vi "Rotating Vectors.vi"() -> ()   [LabVIEW 2015]
uses:
  <vilib>/Analysis/1siggen.llb/Ramp Pattern by Samples.vi
  <vilib>/Analysis/2dsp.llb/Complex FFT.vi
  <vilib>/Analysis/2dsp.llb/Real FFT.vi
  Sub - Arrow Point Calculate.vi
  <vilib>/Analysis/NI_AALPro.lvlib
  <vilib>/Analysis/NI_AALBase.lvlib
panel:
  in  "Message Amplitude":dbl=0.5
  in  "DC Offset":dbl
  in  "RF Frequency":dbl
  in  "Message Frequency":dbl=0.2 step=0.1
  in  "stop":bool
  in  "vi path":path
  in  "Vertical Load Button":bool
  in  "Vertical Pause Button":bool
  in  "Upconvert Baseband":bool=TRUE
  out "Vector Graph":cluster{"z vector":cdb[]}[](graph)=[{"z vector"=[0.0+0.0i, 0.20656463842372266-0.4553361946439979i, 0.21632021300842424-0.355813188436778i, 0.20656463842372266-0.4553361946439979i, 0.12525297407962463-0.3971261161215226i, 0.20656463842372266-0.4553361946439979i]}, {"z vector"=[0.0+0.0i, 0.20656463842372266+0.4553361946439979i, 0.1252529740796247+0.3971261161215225i, 0.20656463842372266+0.4553361946439979i, 0.21632021300842427+0.355813188436778i, 0.20656463842372266+0.4553361946439979i]}, {"z vector"=[0.0+0.0i, 0.4131292768474453+0.0i, 0.32652673646900143+0.05000000000000002i, 0.4131292768474453+0.0i, 0.3265267364690015-0.050000000000000044i, 0.4131292768474453+0.0i]}, {"z vector"=[0.0+0.0i, 0.0+0.0i, nan+nani, 0.0+0.0i, nan+nani, 0.0+0.0i]}, {"z vector"=[0.0+0.0i, 0.4131292768474453+0.0i, 0.32652673646900143+0.05000000000000002i, 0.4131292768474453+0.0i, 0.3265267364690015-0.050000000000000044i, 0.4131292768474453+0.0i]}, {"z vector"=[0.0+0.0i, 0.4131292768474453+0.0i, 0.32652673646900143+0.05000000000000002i, 0.4131292768474453+0.0i, 0.3265267364690015-0.050000000000000044i, 0.4131292768474453+0.0i]}, {"z vector"=[0.4131292768474453+0.0i, 0.4131292768474453+0.0i, nan+nani, 0.4131292768474453+0.0i, nan+nani, 0.4131292768474453+0.0i]}, {"z vector"=[0.0+0.0i, 1.0+0.0i, 0.9133974596215562+0.05000000000000002i, 1.0+0.0i, 0.9133974596215562-0.050000000000000044i, 1.0+0.0i]}]
  out "Time Domain":cluster{dbl, dbl, dbl}(graph)={0.4131292768474453, 0.4131292768474453, 1.0}
  out "Vector Sum Frequency Response":dbl[][](graph)
  out "Individual Vectors":dbl[][](graph)
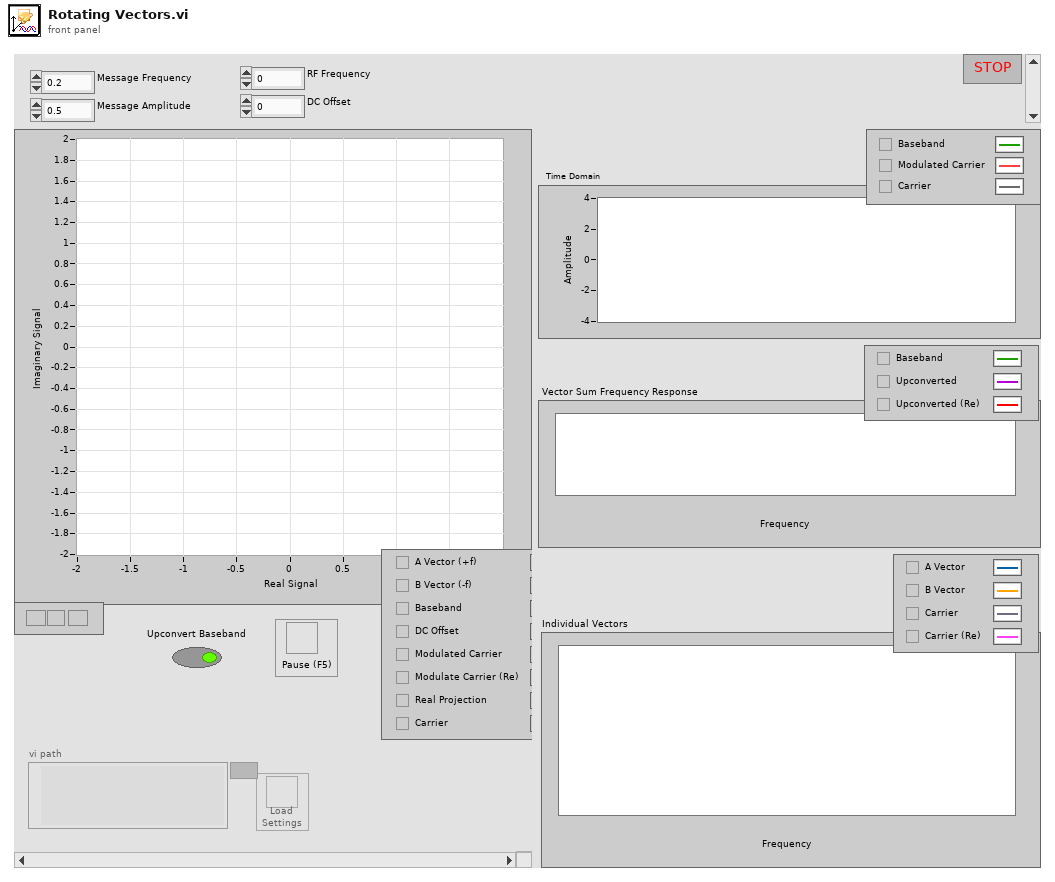
[diagram p1: front panel]
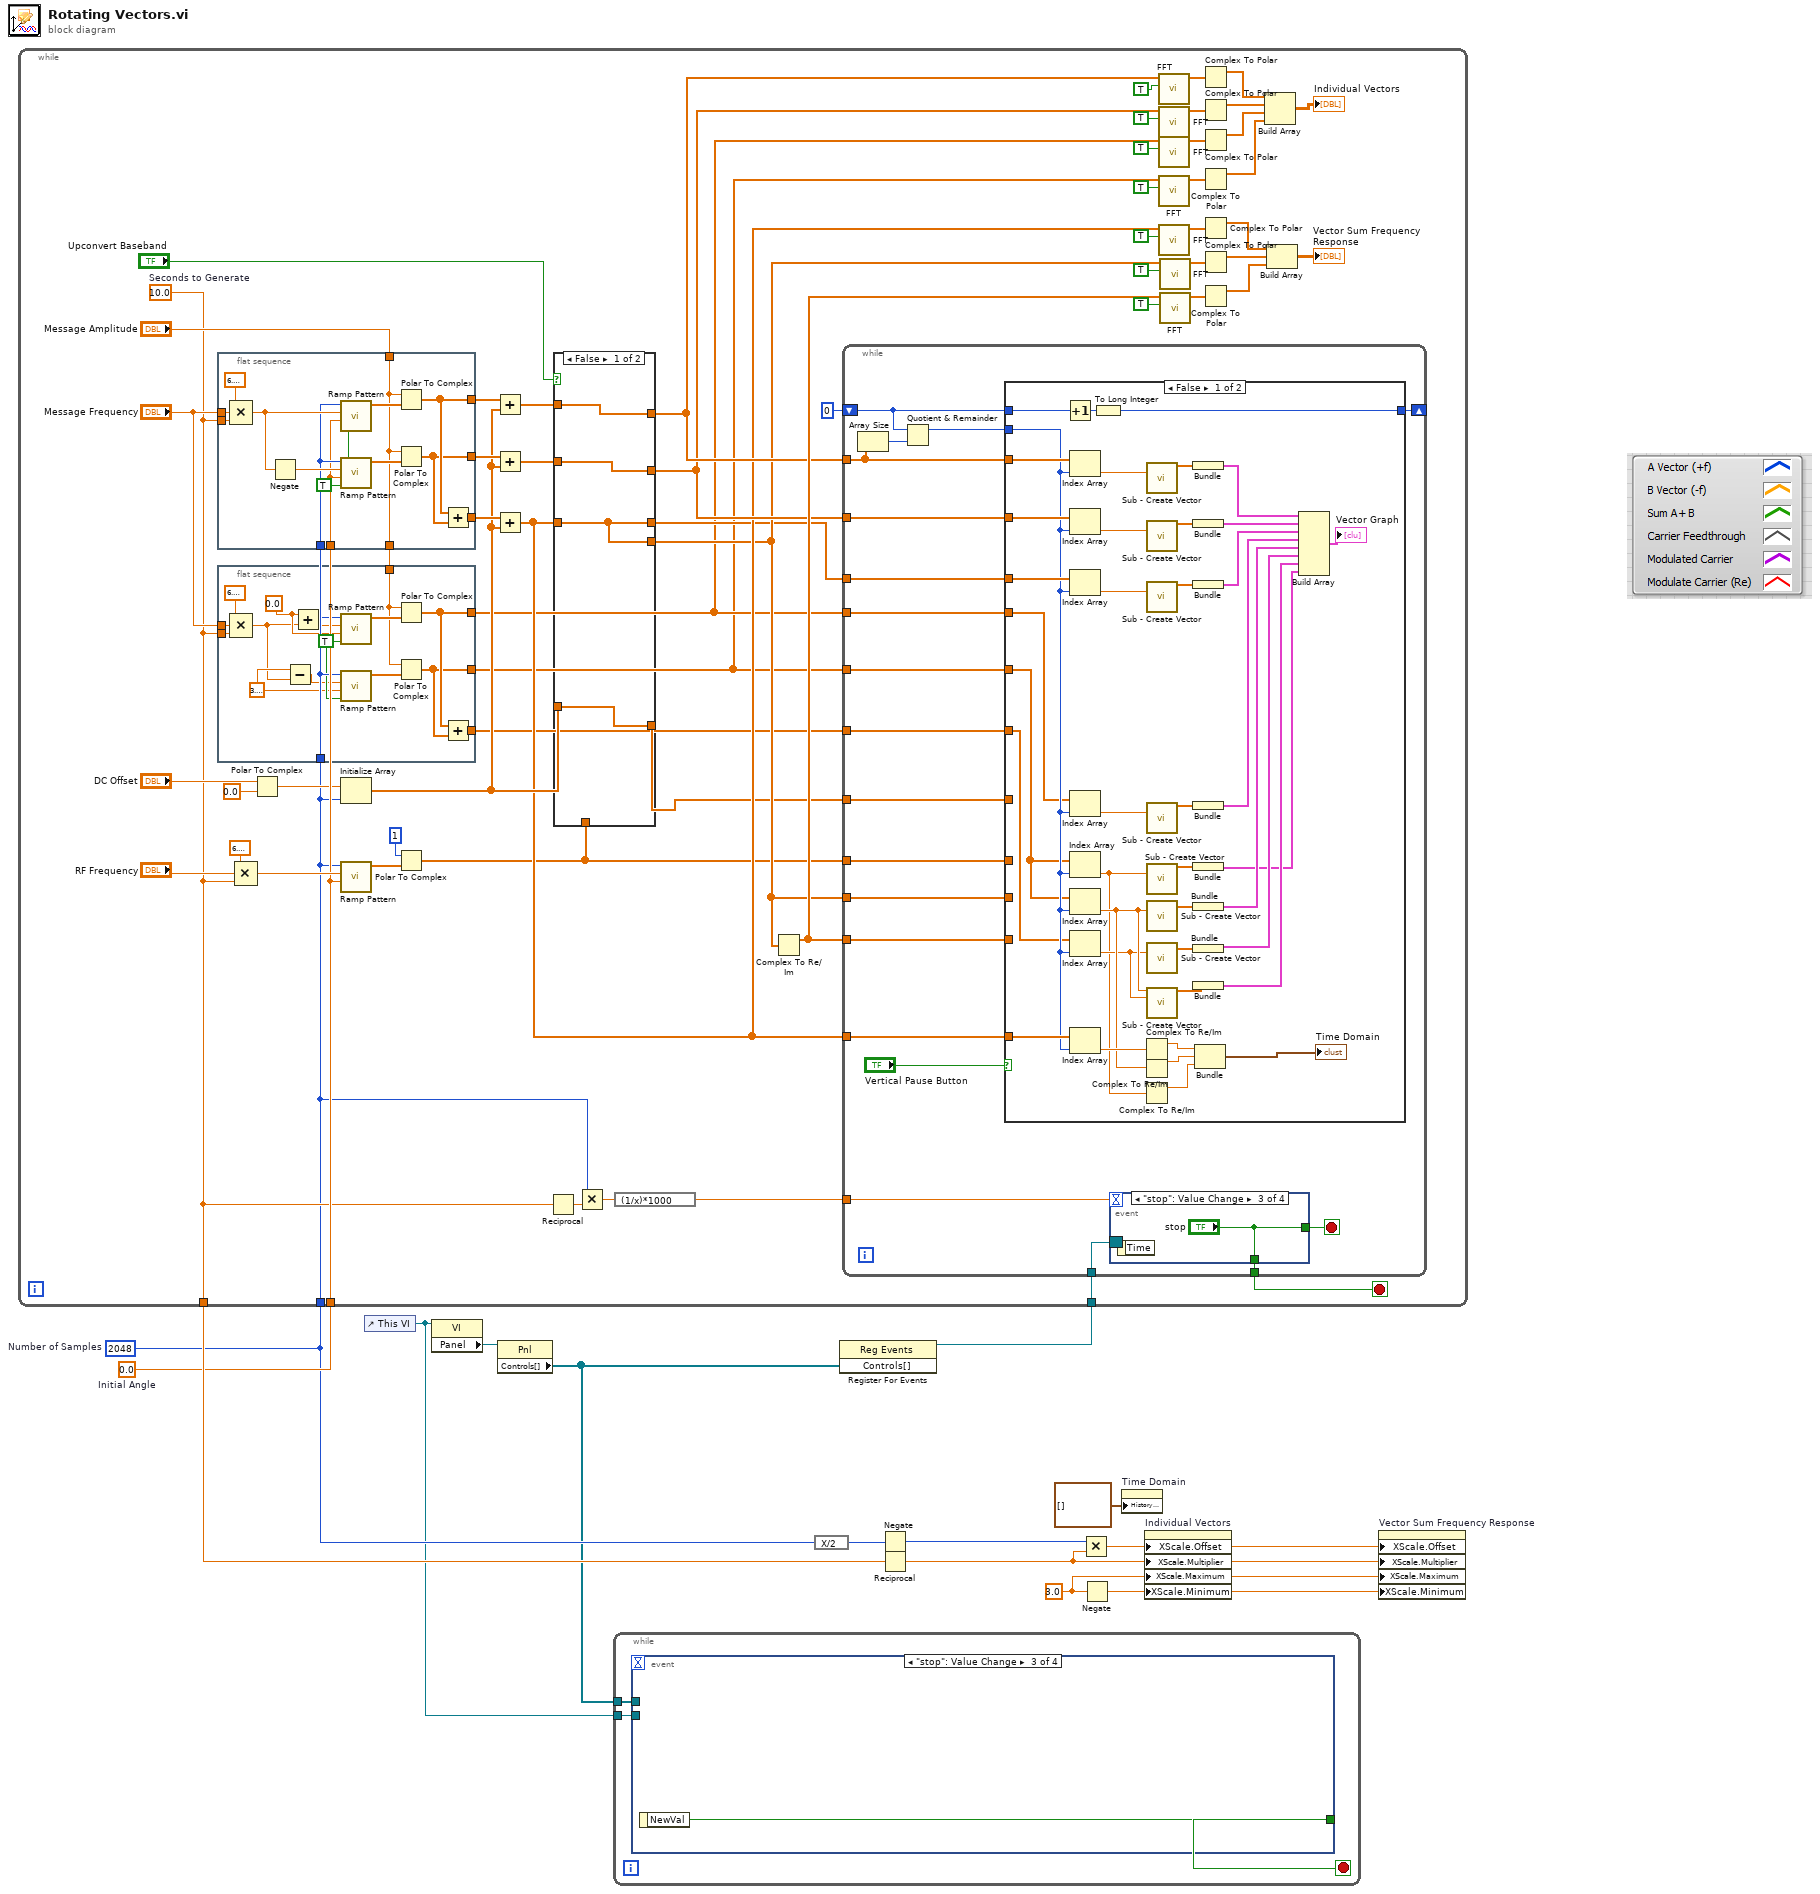
[diagram p0: block diagram]
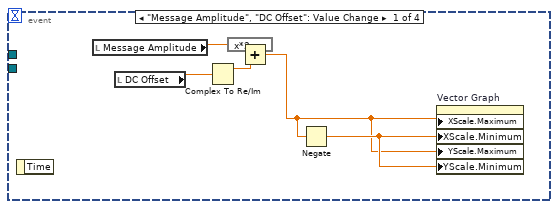
[diagram p2: hidden frame]
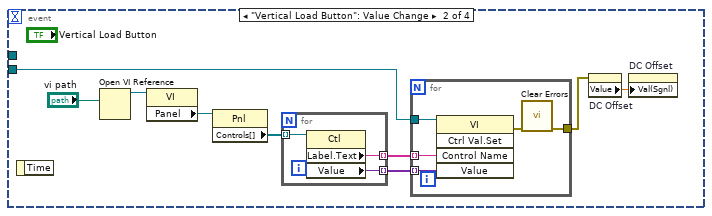
[diagram p3: hidden frame]
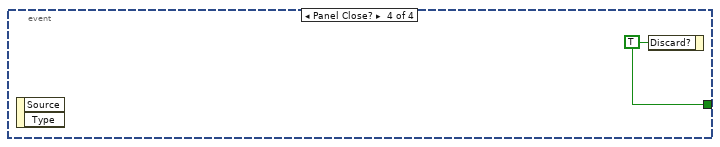
[diagram p4: hidden frame]
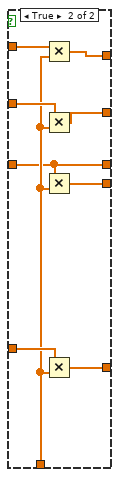
[diagram p5: hidden frame]
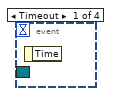
[diagram p7: hidden frame]
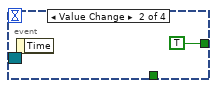
[diagram p8: hidden frame]
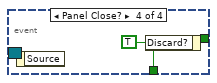
[diagram p9: hidden frame]
diagram:
  w4 = 2048  # Number of Samples
  w5 = 0.0  # Initial Angle
  w11 = 3.0 ("X Scale.Range:Maximum")
  n1 = control-ref of="This VI"() -> (w1:refnum<vi>)
  n2 = property class="VI"(reference=w1) -> ("Panel"=w7:refnum<vi>)  [unwired: 1 in, 2 out]
  n3 = property class="Pnl"(reference=w7) -> ("Controls[]"=w2:refnum<vi>[])  [unwired: 1 in, 2 out]
  n4 = while {
    tunnel: w2 -> [w16]
    tunnel: w1 -> [w15]
    stop <- w17 stop-if-true
    n5 = event shown="[2] \"stop\": Value Change" {
      selector: _ -> [_ _ _ _]
      dyn-events: _ -> [_ _ _ _]
      timeout: _ -> [_ _ _ _]
      tunnel: [_ _ w41 w42] -> w17
      tunnel: w16 -> [_ _ _ _]
      tunnel: w15 -> [_ w29 _ _]
      event "Message Amplitude", "DC Offset": Value Change {
        n6 = event-data() -> ()  [unwired: 1 in, 1 out]
        n7 = local read "Message Amplitude"() -> (w21:dbl)
        n8 = local read "DC Offset"() -> (w22:dbl)
        n9 = Complex To Re/Im(x + iy=w22) -> (x=w19:dbl)  [unwired: 1 out]
        n10 = expression code="x*2"(w21) -> (w18:dbl)
        n11 = Add(x=w18, y=w19) -> (x+y=w20:dbl)
        n12 = Negate(x=w20) -> (-x=w23:dbl)
        n13 = property on="Vector Graph" class="XYGraph (strict)"("XScale.Maximum"=w20, "XScale.Minimum"=w23, "YScale.Maximum"=w20, "YScale.Minimum"=w23) -> ()  [unwired: 2 in, 2 out]
      }
      event "Vertical Load Button": Value Change {
        n14 = event-data() -> ()  [unwired: 1 in, 1 out]
        n15 = Open VI Reference(vi path="vi path") -> (vi reference=w31:refnum<vi>)  [unwired: 5 in, 1 out]
        n16 = property class="VI"(reference=w31) -> ("Panel"=w32:refnum<vi>)  [unwired: 1 in, 2 out]
        n17 = property class="Pnl"(reference=w32) -> ("Controls[]"=w30:refnum<vi>[])  [unwired: 1 in, 2 out]
        n18 = for {
          tunnel: w30 -> [w40] mode=indexing
          tunnel: [w39] -> w28 mode=indexing
          tunnel: [w38] -> w27 mode=indexing
          n19 = property class="Ctl"(reference=w40) -> ("Label.Text"=w39:string, "Value"=w38:variant)  [unwired: 1 in, 2 out]
        }
        n20 = for {
          tunnel: w29 -> [w37]
          tunnel: w28 -> [w36] mode=indexing
          tunnel: w27 -> [w35] mode=indexing
          tunnel: [w33] -> w24
          n21 = invoke class="VI" method="Ctrl Val.Set"(reference=w37, "Control Name"=w36, "Value"=w35) -> (error out=w34:errorcluster)  [unwired: 2 in, 4 out]
          n22 = call <vilib>:"Clear Errors.vi"("error in (no error)"=w34) -> ("error out"=w33:errorcluster)  [unwired: 5 in, 1 out]
        }
        n23 = property on="DC Offset" class="DigNum (strict)"(error in=w24) -> ("Value"=w25:dbl)  [unwired: 1 in, 2 out]
        n24 = property on="DC Offset" class="DigNum (strict)"("Val(Sgnl)"=w25) -> ()  [unwired: 2 in, 2 out]
      }
      event "stop": Value Change {
        n25 = event-data() -> ("NewVal"=w41:bool)  [unwired: 1 in]
      }
      event Panel Close? {
        w42 = TRUE ("Discard?")
        n26 = event-data() -> ()  [unwired: 1 in, 2 out]
        n27 = event-data("Discard?"=w42) -> ()  [unwired: 1 in, 1 out]
      }
    }
  }
  n28 = expression code="X/2"(w4) -> (w13:i32)
  n29 = register-events(w2) -> (reference out=w6:refnum<event-registration>)  [unwired: 2 in, 1 out]
  n30 = while {
    tunnel: [w49] -> w8
    tunnel: w4 -> [w48]
    tunnel: w6 -> [w81]
    tunnel: w5 -> [w72]
    stop <- w79 stop-if-true
    w49 = 10.0  # Seconds to Generate
    n31 = flat-sequence {
      tunnel: "Message Frequency" -> [w132]
      tunnel: [w127] -> w83
      tunnel: [w126] -> w82
      tunnel: w48 -> [w125]
      tunnel: "Message Amplitude" -> [w121]
      tunnel: w49 -> [w124]
      tunnel: [w123] -> w73
      tunnel: w72 -> [w122]
      tunnel: [w121] -> w46
      frame #0 {
        w120 = TRUE ("exclude end?")
        n32 = Compound Arithmetic op=MULTIPLY(6.283185307179586, w132, w124) -> (w128:dbl)
        n33 = Negate(x=w128) -> (-x=w129:dbl)
        n34 = call-poly <vilib>:"Ramp Pattern.vi"("exclude end?"=w120, "start"=w122, "end"=w128, "samples"=w125) -> ("Ramp Pattern"=w131:dbl[])  [unwired: 6 in, 1 out]
        n35 = call-poly <vilib>:"Ramp Pattern.vi"("exclude end?"=w120, "start"=w122, "end"=w129, "samples"=w125) -> ("Ramp Pattern"=w130:dbl[])  [unwired: 6 in, 1 out]
        n36 = Polar To Complex(1:w131, 2:w121) -> (0:w127:cdb[])
        n37 = Polar To Complex(1:w130, 2:w121) -> (0:w126:cdb[])
        n38 = Add(x=w127, y=w126) -> (x+y=w123:cdb[])
      }
    }
    n39 = flat-sequence {
      tunnel: [w116] -> w44
      tunnel: [w115] -> w43
      tunnel: w49 -> [w114]
      tunnel: [w113] -> w47
      tunnel: "Message Frequency" -> [w112]
      tunnel: w48 -> [w111]
      tunnel: w46 -> [w110]
      frame #0 {
        w106 = 3.141592653589793
        w107 = 0.0 ("start")
        w109 = TRUE ("exclude end?")
        n40 = Compound Arithmetic op=MULTIPLY(6.283185307179586, w112, w114) -> (w105:dbl)
        n41 = Subtract(x=w106, y=w105) -> (x-y=w104:dbl)
        n42 = Add(x=w107, y=w105) -> (x+y=w108:dbl)
        n43 = call-poly <vilib>:"Ramp Pattern.vi"("exclude end?"=w109, "start"=w107, "end"=w108, "samples"=w111) -> ("Ramp Pattern"=w118:dbl[])  [unwired: 6 in, 1 out]
        n44 = call-poly <vilib>:"Ramp Pattern.vi"("exclude end?"=w109, "start"=w106, "end"=w104, "samples"=w111) -> ("Ramp Pattern"=w117:dbl[])  [unwired: 6 in, 1 out]
        n45 = Polar To Complex(1:w118, 2:w110) -> (0:w116:cdb[])
        n46 = Polar To Complex(1:w117, 2:w110) -> (0:w115:cdb[])
        n47 = Add(x=w116, y=w115) -> (x+y=w113:cdb[])
      }
    }
    n48 = Compound Arithmetic op=MULTIPLY(6.283185307179586, "RF Frequency", w49) -> (w84:dbl)
    n49 = Polar To Complex(1:0.0 ("theta"), 2:"DC Offset") -> (0:w58:cdb)
    n50 = Initialize Array(w58, w48) -> (w62:cdb[])
    n51 = call-poly <vilib>:"Ramp Pattern.vi"("start"=w72, "end"=w84, "samples"=w48) -> ("Ramp Pattern"=w90:dbl[])  [unwired: 7 in, 1 out]
    n52 = Polar To Complex(1:w90, 2:1) -> (0:w52:cdb[])
    n53 = Add(x=w83, y=w62) -> (x+y=w67:cdb[])
    n54 = Add(x=w82, y=w62) -> (x+y=w66:cdb[])
    n55 = Add(x=w73, y=w62) -> (x+y=w61:cdb[])
    n56 = Reciprocal(x=w49) -> (1/x=w98:dbl)
    n57 = case shown="False" "Upconvert Baseband" {
      tunnel: w67 -> [w135 w146]
      tunnel: w66 -> [w136 w145]
      tunnel: w62 -> [w137 w144]
      tunnel: w61 -> [w134 w138]
      tunnel: w52 -> [_ w143]
      tunnel: [w137 w142] -> w55
      tunnel: [w134 w141] -> w60
      tunnel: [w136 w140] -> w63
      tunnel: [w135 w139] -> w64
      tunnel: [w134 w138] -> w56
      frame False {
      }
      frame True {
        n58 = Multiply(x=w146, y=w143) -> (x*y=w139:cdb[])
        n59 = Multiply(x=w145, y=w143) -> (x*y=w140:cdb[])
        n60 = Multiply(x=w138, y=w143) -> (x*y=w141:cdb[])
        n61 = Multiply(x=w144, y=w143) -> (x*y=w142:cdb[])
      }
    }
    n62 = Multiply(x=w48, y=w98) -> (x*y=w99:dbl)
    n63 = expression code="(1/x)*1000"(w99) -> (w103:dbl)
    n64 = Complex To Re/Im(x + iy=w60) -> (x=w68:dbl[])  [unwired: 1 out]
    n65 = while {
      tunnel: w64 -> [w157]
      tunnel: w103 -> [w162]
      tunnel: w63 -> [w166]
      tunnel: w56 -> [w165]
      tunnel: w60 -> [w164]
      tunnel: w55 -> [w163]
      tunnel: w81 -> [w158]
      tunnel: [w160] -> w79
      tunnel: w68 -> [w159]
      tunnel: w61 -> [w155]
      shift-right: [w152] -> _
      shift-left: 0 -> [w153]
      tunnel: w52 -> [w150]
      tunnel: w44 -> [w149]
      tunnel: w43 -> [w148]
      tunnel: w47 -> [w147]
      stop <- w161 stop-if-true
      n66 = Array Size(array=w157) -> (size(s)=w156:i32)
      n67 = Quotient & Remainder(x=w153, y=w156) -> (x-y*floor(x/y)=w154:i32)  [unwired: 1 out]
      n68 = case shown="False" "Vertical Pause Button" {
        tunnel: w166 -> [w203 _]
        tunnel: w165 -> [w198 _]
        tunnel: w164 -> [_ _]
        tunnel: w163 -> [_ _]
        tunnel: w159 -> [_ _]
        tunnel: w157 -> [w190 _]
        tunnel: w155 -> [w185 _]
        tunnel: w154 -> [w172 _]
        tunnel: w153 -> [w181 w207]
        tunnel: [w180 w207] -> w152
        tunnel: w150 -> [_ _]
        tunnel: w149 -> [w169 _]
        tunnel: w148 -> [w167 _]
        tunnel: w147 -> [w168 _]
        frame False {
          n69 = Increment(x=w181) -> (x+1=w179:i32)
          n70 = Index Array(array=w190, index=w172) -> (element=w187:cdb)
          n71 = Index Array(array=w203, index=w172) -> (element=w188:cdb)
          n72 = Index Array(array=w198, index=w172) -> (element=w189:cdb)
          n73 = Index Array(array=w169, index=w172) -> (element=w186:cdb)
          n74 = Index Array(array=w167, index=w172) -> (element=w171:cdb)
          n75 = Index Array(array=w167, index=w172) -> (element=w176:cdb)
          n76 = Index Array(array=w168, index=w172) -> (element=w175:cdb)
          n77 = Index Array(array=w185, index=w172) -> (element=w184:cdb)
          n78 = To Long Integer(number=w179) -> (32bit integer=w180:i32)
          n79 = Complex To Re/Im(x + iy=w184) -> (x=w197:dbl)  [unwired: 1 out]
          n80 = Complex To Re/Im(x + iy=w176) -> (x=w196:dbl)  [unwired: 1 out]
          n81 = Complex To Re/Im(x + iy=w171) -> (x=w170:dbl)  [unwired: 1 out]
          n82 = call "Sub - Create Vector.vi"("Vector End"=w187) -> ("Vector Points"=w202:cdb[])  [unwired: 14 in]
          n83 = call "Sub - Create Vector.vi"("Vector End"=w188) -> ("Vector Points"=w201:cdb[])  [unwired: 14 in]
          n84 = call "Sub - Create Vector.vi"("Vector End"=w189) -> ("Vector Points"=w199:cdb[])  [unwired: 14 in]
          n85 = call "Sub - Create Vector.vi"("Vector End"=w186) -> ("Vector Points"=w194:cdb[])  [unwired: 14 in]
          n86 = call "Sub - Create Vector.vi"("Vector End"=w171) -> ("Vector Points"=w174:cdb[])  [unwired: 14 in]
          n87 = call "Sub - Create Vector.vi"("Vector End"=w176) -> ("Vector Points"=w192:cdb[])  [unwired: 14 in]
          n88 = call "Sub - Create Vector.vi"("Vector End"=w175) -> ("Vector Points"=w191:cdb[])  [unwired: 14 in]
          n89 = call "Sub - Create Vector.vi"("Vector Start (0 +0i)"=w176, "Vector End"=w175) -> ("Vector Points"=w178:cdb[])  [unwired: 13 in]
          n90 = Bundle("Vector Points"=w202) -> (w206:cluster{"Vector Points":cdb[]})  [unwired: 1 in]
          n91 = Bundle("Vector Points"=w201) -> (w204:cluster{"Vector Points":cdb[]})  [unwired: 1 in]
          n92 = Bundle("Vector Points"=w199) -> (w200:cluster{"Vector Points":cdb[]})  [unwired: 1 in]
          n93 = Bundle("Vector Points"=w194) -> (w193:cluster{"Vector Points":cdb[]})  [unwired: 1 in]
          n94 = Bundle("Vector Points"=w174) -> (w173:cluster{"Vector Points":cdb[]})  [unwired: 1 in]
          n95 = Bundle("Vector Points"=w192) -> (w183:cluster{"Vector Points":cdb[]})  [unwired: 1 in]
          n96 = Bundle("Vector Points"=w191) -> (w182:cluster{"Vector Points":cdb[]})  [unwired: 1 in]
          n97 = Bundle("Vector Points"=w178) -> (w177:cluster{"Vector Points":cdb[]})  [unwired: 1 in]
          n98 = Bundle(w197, w196, w170) -> (→"Time Domain":cluster{dbl, dbl, dbl})  [unwired: 1 in]
          n99 = Build Array(w206, w204, w200, w193, w183, w182, w177, w173) -> (→"Vector Graph":cluster{"Vector Points":cdb[]}[])
        }
        frame True {
        }
      }
      n100 = event shown="[2] \"stop\": Value Change" {
        selector: w158 -> [_ _ _ _]
        dyn-events: _ -> [_ _ _ _]
        timeout: w162 -> [_ _ _ _]
        tunnel: [_ TRUE "stop" w210] -> w161
        tunnel: [_ _ "stop" w210] -> w160
        event Timeout {
          n101 = event-data() -> ()  [unwired: 1 in, 1 out]
        }
        event Value Change {
          n102 = event-data() -> ()  [unwired: 1 in, 1 out]
        }
        event "stop": Value Change {
          n103 = event-data() -> ()  [unwired: 1 in, 1 out]
        }
        event Panel Close? {
          w210 = TRUE ("Discard?")
          n104 = event-data() -> ()  [unwired: 1 in, 1 out]
          n105 = event-data("Discard?"=w210) -> ()  [unwired: 1 in, 1 out]
        }
      }
    }
    n106 = call-poly <vilib>:"FFT.vi"("shift?"=TRUE, "X"=w64) -> ("FFT {X}"=w101:cdb[])  [unwired: 8 in, 1 out]
    n107 = call-poly <vilib>:"FFT.vi"("shift?"=TRUE, "X"=w63) -> ("FFT {X}"=w97:cdb[])  [unwired: 8 in, 1 out]
    n108 = call-poly <vilib>:"FFT.vi"("shift?"=TRUE, "X"=w44) -> ("FFT {X}"=w76:cdb[])  [unwired: 8 in, 1 out]
    n109 = call-poly <vilib>:"FFT.vi"("shift?"=TRUE, "X"=w43) -> ("FFT {X}"=w54:cdb[])  [unwired: 8 in, 1 out]
    n110 = call-poly <vilib>:"FFT.vi"("shift?"=TRUE, "X"=w61) -> ("FFT {X}"=w92:cdb[])  [unwired: 8 in, 1 out]
    n111 = call-poly <vilib>:"FFT.vi"("shift?"=TRUE, "X"=w60) -> ("FFT {X}"=w88:cdb[])  [unwired: 8 in, 1 out]
    n112 = call-poly <vilib>:"FFT.vi"("shift?"=TRUE, "X"=w68) -> ("FFT {X}"=w70:cdb[])  [unwired: 8 in, 1 out]
    n113 = Complex To Polar(r * e^(i*theta)=w101) -> (r=w100:dbl[])  [unwired: 1 out]
    n114 = Complex To Polar(r * e^(i*theta)=w97) -> (r=w94:dbl[])  [unwired: 1 out]
    n115 = Complex To Polar(r * e^(i*theta)=w76) -> (r=w75:dbl[])  [unwired: 1 out]
    n116 = Complex To Polar(r * e^(i*theta)=w54) -> (r=w51:dbl[])  [unwired: 1 out]
    n117 = Complex To Polar(r * e^(i*theta)=w92) -> (r=w91:dbl[])  [unwired: 1 out]
    n118 = Complex To Polar(r * e^(i*theta)=w88) -> (r=w86:dbl[])  [unwired: 1 out]
    n119 = Complex To Polar(r * e^(i*theta)=w70) -> (r=w69:dbl[])  [unwired: 1 out]
    n120 = Build Array(w100, w94, w75, w51) -> (→"Individual Vectors":dbl[][])
    n121 = Build Array(w91, w86, w69) -> (→"Vector Sum Frequency Response":dbl[][])
  }
  n122 = Negate(x=w13) -> (-x=w14:i32)
  n123 = Reciprocal(x=w8) -> (1/x=w10:dbl)
  n124 = Multiply(x=w14, y=w10) -> (x*y=w9:dbl)
  n125 = Negate(x=w11) -> (-x=w12:dbl)
  n126 = property on="Time Domain" class="WFChart (strict)"("History Data"=cluster{dbl, dbl, dbl}[] []) -> ()  [unwired: 2 in, 2 out]
  n127 = property on="Individual Vectors" class="WFGraph (strict)"("XScale.Offset"=w9, "XScale.Multiplier"=w10, "XScale.Maximum"=w11, "XScale.Minimum"=w12) -> ()  [unwired: 2 in, 2 out]
  n128 = property on="Vector Sum Frequency Response" class="WFGraph (strict)"("XScale.Offset"=w9, "XScale.Multiplier"=w10, "XScale.Maximum"=w11, "XScale.Minimum"=w12) -> ()  [unwired: 2 in, 2 out]
